vi "Close.vi"(8 "error in (no error)":errorcluster, 11 "Refnum":refnum<k7>) -> (0 "error out":errorcluster)   [LabVIEW 2020, in "lvpptx.lvlib"]
uses:
  lvpptx.lvlib
panel:
  # "Quit and close connection.\nIf you want to keep the PPT window open, just close the refnum"
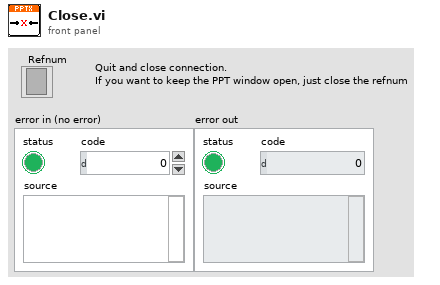
[diagram p1: front panel]
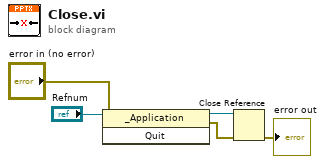
[diagram p0: block diagram]
diagram:
  n1 = invoke class="_Application" method="Quit"(reference="Refnum", error in="error in (no error)") -> (reference out=w4:refnum<k7>, error out=w3:errorcluster)  [unwired: 1 in, 1 out]
  n2 = Close Reference(reference=w4, error in (no error)=w3) -> (error out=→"error out":errorcluster)
